vi "test_Create (JSON RCT).vi"(8 "error in":errorcluster) -> (0 "error out":errorcluster)   [LabVIEW 2020, in "Test_Routing Templates.lvlib"]
uses:
  Test_Routing Templates.lvlib
  <vilib>/addons/_JKI Toolkits/Caraya/classes/Assert/Assert Not Error.vi
  <vilib>/addons/_JKI Toolkits/Caraya/classes/Assert/Assert Error.vi
  <vilib>/addons/_JKI Toolkits/Caraya/classes/Test/Test.lvclass
  <vilib>/addons/_JKI Toolkits/Caraya/classes/Assert/Assert.lvclass
  Routing Channel Templates/JSON Routing Channel Template/JSON Routing Channel Template.lvclass
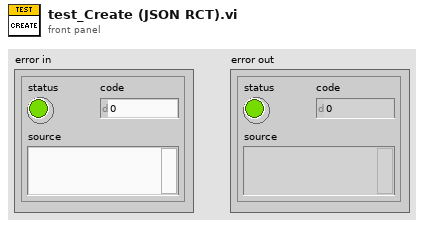
[diagram p1: front panel]
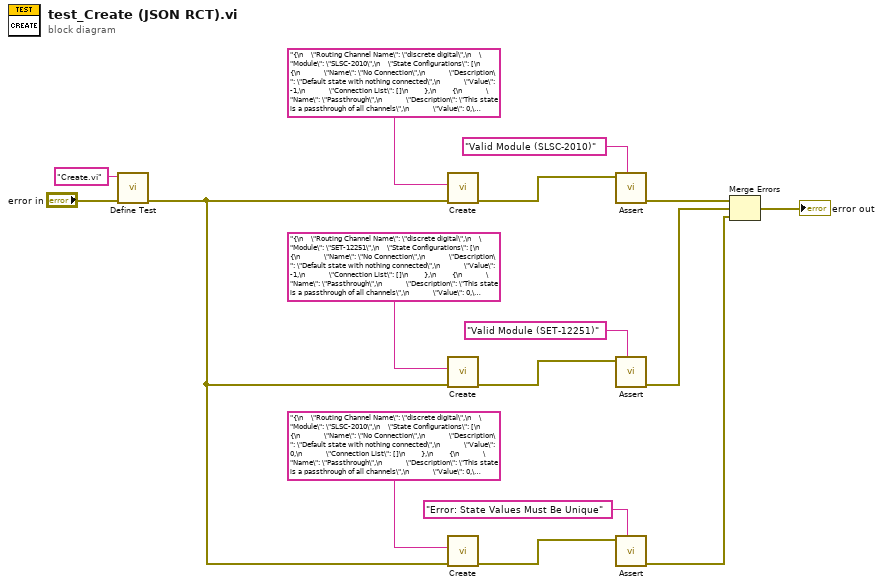
[diagram p0: block diagram]
diagram:
  n1 = call <vilib>:"Define Test.vi"("error in (no error)"="error in", "Label (VI Title)"="Create.vi") -> ("error out"=w1:errorcluster)  [unwired: 9 in]
  n2 = call "Create.vi"("error in (no error)"=w1, "JSON"="{\n    \"Routing Channel Name\": \"discrete digital\",\n    \"Module\": \"SLSC-2010\",\n    \"State Configurations\": [\n        {\n            \"Name\": \"No Connection\",\n            \"Description\": \"Default state with nothing connected\",\n            \"Value\": -1,\n            \"Connection List\": []\n        },\n        {\n            \"Name\": \"Passthrough\",\n            \"Description\": \"This state is a passthrough of all channels\",\n            \"Value\": 0,\n            \"Connection List\": [\n                {\n                    \"Channel\": \"DI+\",\n                    \"Connection Type\": \"Passthrough\"\n                },\n                {\n                    \"Channel\": \"DI-\",\n                    \"Connection Type\": \"Passthrough\"\n                }\n            ]\n        },\n        {\n            \"Name\": \"Real-Sim\",\n            \"Description\": \"Connect J1 to J2 pins\",\n            \"Value\": 1,\n            \"Connection List\": [\n                {\n                    \"Channel\": \"DI+\",\n                    \"Connection Type\": \"Real-Sim\"\n                },\n                {\n                    \"Channel\": \"DI-\",\n                    \"Connection Type\": \"Real-Sim\"\n                }\n            ]\n        }\n    ]\n}" ("text")) -> ("error out"=w12:errorcluster)  [unwired: 8 in, 1 out]
  n3 = call "Create.vi"("error in (no error)"=w1, "JSON"="{\n    \"Routing Channel Name\": \"discrete digital\",\n    \"Module\": \"SET-12251\",\n    \"State Configurations\": [\n        {\n            \"Name\": \"No Connection\",\n            \"Description\": \"Default state with nothing connected\",\n            \"Value\": -1,\n            \"Connection List\": []\n        },\n        {\n            \"Name\": \"Passthrough\",\n            \"Description\": \"This state is a passthrough of all channels\",\n            \"Value\": 0,\n            \"Connection List\": [\n                {\n                    \"Channel\": \"DI+\",\n                    \"Connection Type\": \"Passthrough\"\n                },\n                {\n                    \"Channel\": \"DI-\",\n                    \"Connection Type\": \"Passthrough\"\n                }\n            ]\n        },\n        {\n            \"Name\": \"Real-Sim\",\n            \"Description\": \"Connect J1 to J2 pins\",\n            \"Value\": 1,\n            \"Connection List\": [\n                {\n                    \"Channel\": \"DI+\",\n                    \"Connection Type\": \"Real-Sim\"\n                },\n                {\n                    \"Channel\": \"DI-\",\n                    \"Connection Type\": \"Real-Sim\"\n                }\n            ]\n        }\n    ]\n}" ("text")) -> ("error out"=w8:errorcluster)  [unwired: 8 in, 1 out]
  n4 = call "Create.vi"("error in (no error)"=w1, "JSON"="{\n    \"Routing Channel Name\": \"discrete digital\",\n    \"Module\": \"SLSC-2010\",\n    \"State Configurations\": [\n        {\n            \"Name\": \"No Connection\",\n            \"Description\": \"Default state with nothing connected\",\n            \"Value\": 0,\n            \"Connection List\": []\n        },\n        {\n            \"Name\": \"Passthrough\",\n            \"Description\": \"This state is a passthrough of all channels\",\n            \"Value\": 0,\n            \"Connection List\": [\n                {\n                    \"Channel\": \"DI+\",\n                    \"Connection Type\": \"Passthrough\"\n                },\n                {\n                    \"Channel\": \"DI-\",\n                    \"Connection Type\": \"Passthrough\"\n                }\n            ]\n        },\n        {\n            \"Name\": \"Real-Sim\",\n            \"Description\": \"Connect J1 to J2 pins\",\n            \"Value\": 1,\n            \"Connection List\": [\n                {\n                    \"Channel\": \"DI+\",\n                    \"Connection Type\": \"Real-Sim\"\n                },\n                {\n                    \"Channel\": \"DI-\",\n                    \"Connection Type\": \"Real-Sim\"\n                }\n            ]\n        }\n    ]\n}" ("text")) -> ("error out"=w4:errorcluster)  [unwired: 8 in, 1 out]
  n5 = call-poly <vilib>:"Assert.vi"("Label"="Valid Module (SLSC-2010)", "Not Error?"=w12) -> ("error out"=w14:errorcluster)  [unwired: 9 in]
  n6 = call-poly <vilib>:"Assert.vi"("Label"="Valid Module (SET-12251)", "Error?"=w8) -> ("error out"=w6:errorcluster)  [unwired: 9 in]
  n7 = call-poly <vilib>:"Assert.vi"("Label"="Error: State Values Must Be Unique", "Error?"=w4) -> ("error out"=w2:errorcluster)  [unwired: 9 in]
  n8 = Merge Errors(w14, w6, w2) -> (→"error out":errorcluster)
